vi "Init Command.vi"(5 "Sequencer":refnum<class "MessageQ.lvclass">, 6 "Variables":refnum<class "Variables.lvclass">, 7 "VolatusAPI":refnum<class "VolatusAPI.lvclass">, 8 "error in (no error)":refnum<class "MultiErrors.lvclass">, 10 "Command Config":refnum<class "Command Config.lvclass">, 11 "Start Log Command in":refnum<class "Start Log Command.lvclass">) -> (0 "error out":refnum<class "MultiErrors.lvclass">, 3 "Start Log Command out":T1)   [LabVIEW 2020, in "VolatusSeq.lvlib" / "Start Log Command.lvclass"]
uses:
  Start Log Command.lvclass
  VolatusErrorUtilities/MultiErrors/MultiErrors.lvclass
  Command.ctl
  Volatus/MessageQ/MessageQ.lvclass
  VolatusSeqConfig/Command Type.ctl
  messages/CmdDigital/Data.ctl
  messages/CmdAnalog/Data.ctl
  Send Type.ctl
  Volatus/VolatusAPI/VolatusAPI.lvclass
  VolatusSeqConfig/Command Config/Command Config.lvclass
  VolatusSeqConfig/Start Log Command Config/Start Log Command Config.lvclass
  Start Log Command.lvclass/Start Log Command.ctl
  VolatusSeqConfig/VolatusSeqConfig.lvlib
  VolatusSeq.lvlib
  messages/CmdAnalog/CmdAnalog.lvlib
  messages/CmdDigital/CmdDigital.lvlib
  Variables/Variables.lvclass
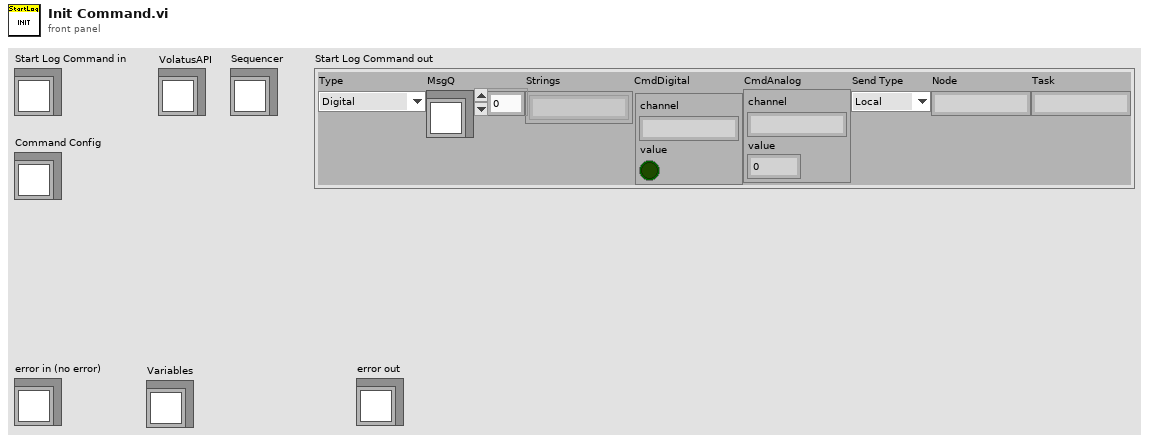
[diagram p1: front panel]
types:
  T1 = typedef "VolatusSeq.lvlib/Command.ctl" = cluster{"Type":T2, "MsgQ":refnum<class "MessageQ.lvclass">, "Strings":string[], "CmdDigital":T3, "CmdAnalog":T4, "Send Type":T5, "Node":string, "Task":string}
  T2 = typedef "VolatusSeqConfig.lvlib/Command Type.ctl" = enum16{"Digital", "Numeric", "Transition", "Stop", "StartLog", "StopLog", "Start", "Event", "Error", "HTTP"}
  T3 = typedef "CmdDigital.lvlib/Data.ctl" = cluster{"channel":string, "value":bool}
  T4 = typedef "CmdAnalog.lvlib/Data.ctl" = cluster{"channel":string, "value":dbl}
  T5 = typedef "VolatusSeq.lvlib/Send Type.ctl" = enum16{"Local", "Remote"}
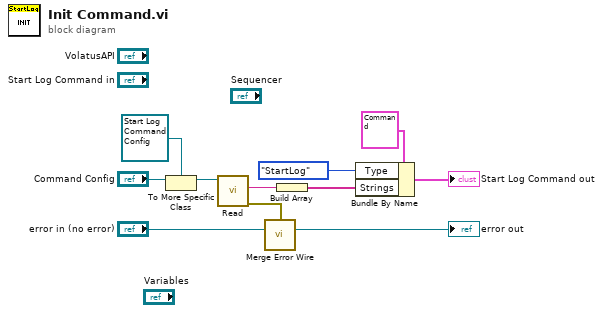
[diagram p0: block diagram]
diagram:
  n1 = To More Specific Class(target class=refnum<class "Start Log Command Config.lvclass"> refnum ("VolatusSeqConfig.lvlib:Start Log Command Config.lvclass"), reference="Command Config") -> (specific class reference=w9:refnum<class "Start Log Command Config.lvclass">)  [unwired: 1 in, 1 out]
  n2 = call "Read.vi"("Start Log Command Config in"=w9) -> ("error out"=w6:errorcluster, "Test"=w3:string)  [unwired: 8 in, 1 out]
  n3 = call "Merge Error Wire.vi"("error in (no error)"=w6, "MultiErrors in"="error in (no error)") -> ("MultiErrors out"=→"error out":refnum<class "MultiErrors.lvclass">)  [unwired: 13 in]
  n4 = Build Array(w3) -> (w2:string[])
  n5 = Bundle By Name(cluster=T1 {"Type"=enum."Digital", "MsgQ"=refnum, "Strings"=[], "CmdDigital"={"channel"="", "value"=FALSE}, "CmdAnalog"={"channel"="", "value"=0.0}, "Send Type"=enum."Local", "Node"="", "Task"=""} ("Start Log Command out"), "Type"=Command_Type."StartLog", "Strings"=w2) -> (→"Start Log Command out":T1)
